vi "Calcualte B Matrix.vi"(6 "Tag ID":i32, 9 "Camera intrinsic matrix (K^-1)":dbl[][](array[numeric]), 10 "Homography H":T1) -> (0 "t Translation Vector":dbl[](array[numeric]), 1 "R Rotation Matrix (final)":T1 format="%#_6f", 2 "B Matrix":dbl[][](array[numeric]))   [LabVIEW 2025]
uses:
  <vilib>/Analysis/Matrix/Datatypes/RealMatrix.ctl
  <vilib>/Analysis/baseanly.llb/Real A x B.vi
  <vilib>/Analysis/baseanly.llb/Real Determinant.vi
  <vilib>/Analysis/7linalg.llb/Real SVD Decomposition.vi
  <vilib>/Analysis/NI_AALPro.lvlib
  <vilib>/Analysis/NI_AALBase.lvlib
  <vilib>/Analysis/Matrix/NI_Matrix.lvlib
panel:
  out "Matrix V":T1
  out "detR":dbl format="%.6f"
  out "detR_temp":dbl format="%.6f"
  out "R^tR":T1 format="%#.3f"
  out "v^t":T1 format="%#_6f"
  out "b1 lambda":dbl
  out "R Matrix":dbl[][](array[numeric])
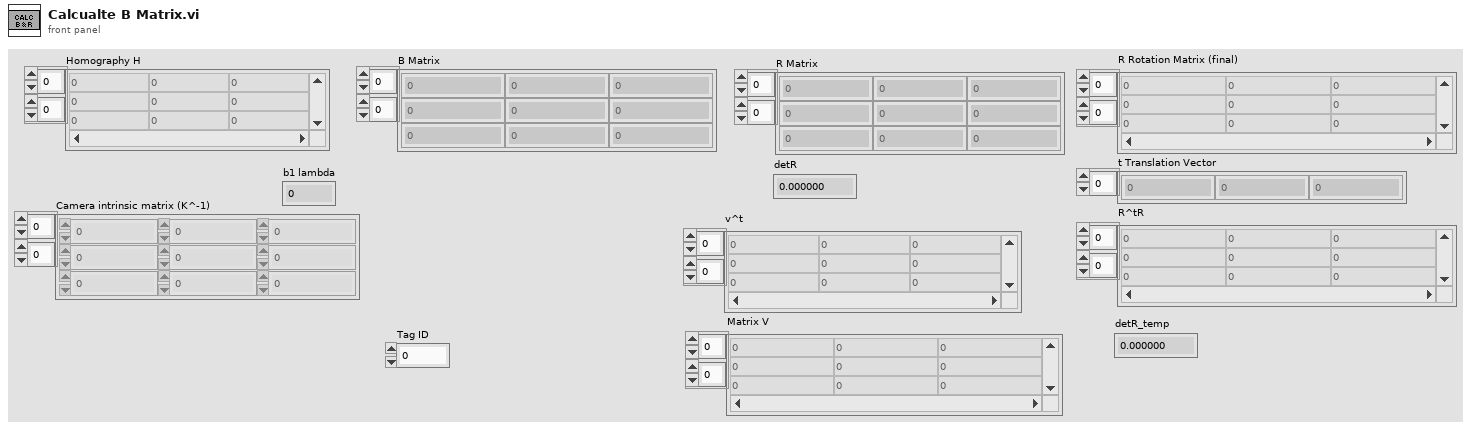
[diagram p1: front panel]
types:
  T1 = typedef "NI_Matrix.lvlib/RealMatrix.ctl" = dbl[][]
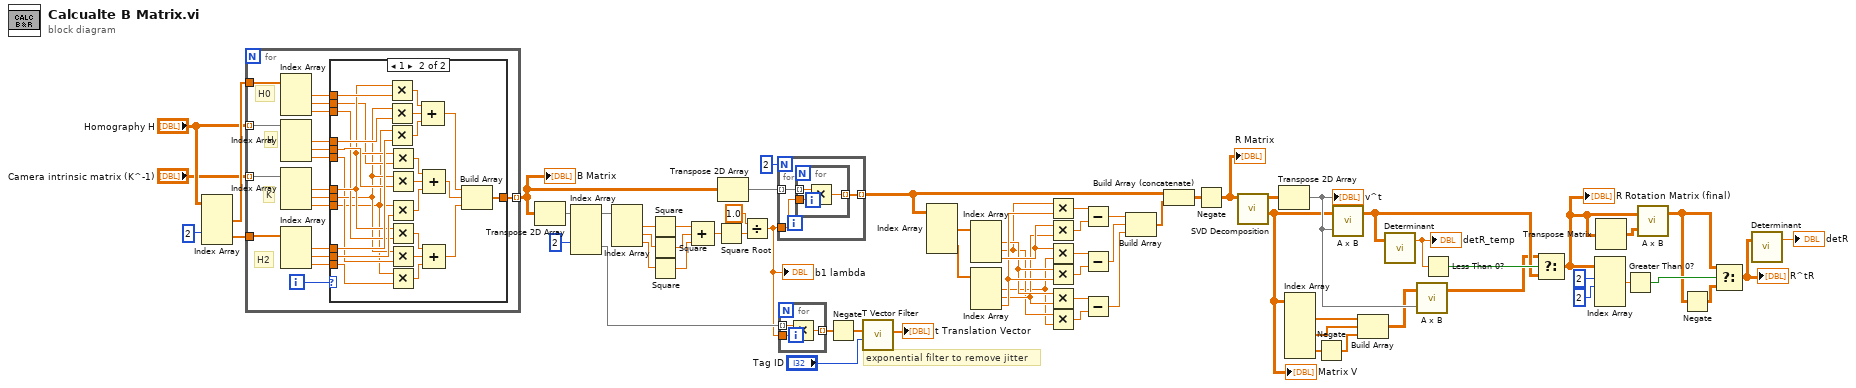
[diagram p0: block diagram]
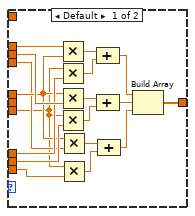
[diagram p2: hidden frame]
diagram:
  # "exponential filter to remove jitter"
  n1 = Index Array(array="Homography H", index (row) #2=2 ("index (row)")) -> (element #1=w69:dbl[], element #2=w68:dbl[])  [unwired: 3 in]
  n2 = for {
    tunnel: "Homography H" -> [w86] mode=indexing
    tunnel: "Camera intrinsic matrix (K^-1)" -> [w87] mode=indexing
    tunnel: w68 -> [w83]
    tunnel: [w76] -> w63 mode=indexing
    tunnel: w69 -> [w73]
    i -> [w75]
    # "H0"
    # "H2"
    # "K"
    # "H"
    n3 = Index Array(array=w73) -> (element #1=w72:dbl, element #2=w71:dbl, element #3=w70:dbl)  [unwired: 3 in]
    n4 = Index Array(array=w86) -> (element #1=w85:dbl, element #2=w84:dbl, element #3=w79:dbl)  [unwired: 3 in]
    n5 = Index Array(array=w87) -> (element #1=w80:dbl, element #2=w74:dbl, element #3=w78:dbl)  [unwired: 3 in]
    n6 = Index Array(array=w83) -> (element #1=w82:dbl, element #2=w81:dbl, element #3=w77:dbl)  [unwired: 3 in]
    n7 = case shown="1" w75 {
      tunnel: w85 -> [w101 w127]
      tunnel: w84 -> [w100 w119]
      tunnel: w82 -> [w99 w125]
      tunnel: w81 -> [w98 w117]
      tunnel: w80 -> [w95 w113]
      tunnel: w79 -> [w94 w108]
      tunnel: w78 -> [w93 w107]
      tunnel: w77 -> [w92 w106]
      tunnel: [w88 w130] -> w76
      tunnel: w74 -> [_ w109]
      tunnel: w72 -> [_ w129]
      tunnel: w71 -> [_ w112]
      tunnel: w70 -> [_ w110]
      frame Default {
        n8 = Multiply(x=w101, y=w95) -> (x*y=w105:dbl)
        n9 = Multiply(x=w93, y=w99) -> (x*y=w104:dbl)
        n10 = Multiply(x=w95, y=w100) -> (x*y=w103:dbl)
        n11 = Multiply(x=w93, y=w98) -> (x*y=w102:dbl)
        n12 = Multiply(x=w95, y=w94) -> (x*y=w96:dbl)
        n13 = Multiply(x=w93, y=w92) -> (x*y=w97:dbl)
        n14 = Compound Arithmetic op=ADD(w105, w104) -> (w91:dbl)
        n15 = Compound Arithmetic op=ADD(w103, w102) -> (w90:dbl)
        n16 = Compound Arithmetic op=ADD(w96, w97) -> (w89:dbl)
        n17 = Build Array(w91, w90, w89) -> (w88:dbl[])
      }
      frame 1 {
        n18 = Multiply(x=w113, y=w129) -> (x*y=w128:dbl)
        n19 = Multiply(x=w109, y=w127) -> (x*y=w126:dbl)
        n20 = Multiply(x=w107, y=w125) -> (x*y=w124:dbl)
        n21 = Multiply(x=w113, y=w112) -> (x*y=w120:dbl)
        n22 = Multiply(x=w109, y=w119) -> (x*y=w121:dbl)
        n23 = Multiply(x=w107, y=w117) -> (x*y=w122:dbl)
        n24 = Multiply(x=w113, y=w110) -> (x*y=w116:dbl)
        n25 = Multiply(x=w109, y=w108) -> (x*y=w115:dbl)
        n26 = Multiply(x=w107, y=w106) -> (x*y=w114:dbl)
        n27 = Compound Arithmetic op=ADD(w128, w126, w124) -> (w123:dbl)
        n28 = Compound Arithmetic op=ADD(w120, w121, w122) -> (w118:dbl)
        n29 = Compound Arithmetic op=ADD(w116, w115, w114) -> (w111:dbl)
        n30 = Build Array(w123, w118, w111) -> (w130:dbl[])
      }
    }
  }
  "B Matrix" <- w63
  n31 = Transpose 2D Array(2D array=w63) -> (transposed array=w64:dbl[][])
  n32 = Index Array(array=w64, index (row) #2=2 ("index (row)")) -> (element #1=w32:dbl[], element #2=w30:dbl[])  [unwired: 3 in]
  n33 = Index Array(array=w32) -> (element #1=w60:dbl, element #2=w59:dbl, element #3=w58:dbl)  [unwired: 3 in]
  n34 = Square(x=w60) -> (x^2=w57:dbl)
  n35 = Square(x=w59) -> (x^2=w56:dbl)
  n36 = Square(x=w58) -> (x^2=w55:dbl)
  n37 = Compound Arithmetic op=ADD(w57, w56, w55) -> (w54:dbl)
  n38 = Square Root(x=w54) -> (sqrt(x)=w52:dbl)
  n39 = Transpose 2D Array(2D array=w63) -> (transposed array=w62:dbl[][])
  n40 = Divide(x=1.0, y=w52) -> (x/y=w29:dbl)
  "b1 lambda" <- w29
  n41 = for {
    N: 2 -> [_]
    tunnel: w62 -> [w133] mode=indexing
    tunnel: w29 -> [w132]
    tunnel: [w131] -> w51 mode=indexing
    n42 = for {
      tunnel: w133 -> [w136] mode=indexing
      tunnel: w132 -> [w135]
      tunnel: [w134] -> w131 mode=indexing
      n43 = Multiply(x=w136, y=w135) -> (x*y=w134:dbl)
    }
  }
  n44 = for {
    tunnel: w30 -> [w138] mode=indexing
    tunnel: w29 -> [w139]
    tunnel: [w137] -> w28 mode=indexing
    n45 = Multiply(x=w138, y=w139) -> (x*y=w137:dbl)
  }
  n46 = Negate(x=w28) -> (-x=w3:dbl[])
  n47 = call "T Vector Filter.vi"("Tag ID"="Tag ID", "t Translation Vector"=w3) -> ("t Translation Vector filtered"=→"t Translation Vector":dbl[])  [unwired: 9 in]
  n48 = Index Array(array=w51) -> (element #1=w50:dbl[], element #2=w49:dbl[])  [unwired: 4 in]
  n49 = Index Array(array=w50) -> (element #1=w40:dbl, element #2=w38:dbl, element #3=w44:dbl)  [unwired: 3 in]
  n50 = Index Array(array=w49) -> (element #1=w37:dbl, element #2=w39:dbl, element #3=w43:dbl)  [unwired: 3 in]
  n51 = Multiply(x=w38, y=w43) -> (x*y=w48:dbl)
  n52 = Multiply(x=w44, y=w39) -> (x*y=w47:dbl)
  n53 = Multiply(x=w44, y=w37) -> (x*y=w45:dbl)
  n54 = Multiply(x=w40, y=w43) -> (x*y=w46:dbl)
  n55 = Multiply(x=w40, y=w39) -> (x*y=w41:dbl)
  n56 = Multiply(x=w38, y=w37) -> (x*y=w42:dbl)
  n57 = Subtract(x=w48, y=w47) -> (x-y=w36:dbl)
  n58 = Subtract(x=w45, y=w46) -> (x-y=w35:dbl)
  n59 = Subtract(x=w41, y=w42) -> (x-y=w34:dbl)
  n60 = Build Array(w36, w35, w34) -> (w33:dbl[])
  n61 = Build Array (concatenate)(w51, w33) -> (w26:dbl[][])
  n62 = Negate(x=w26) -> (-x=w24:dbl[][])
  "R Matrix" <- w24
  n63 = call-poly <vilib>:"SVD Decomposition.vi"("A"=w24) -> ("Matrix V"=w6:T1, "Matrix U"=w27:T1)  [unwired: 6 in, 3 out]
  "Matrix V" <- w6
  n64 = Transpose 2D Array(2D array=w27) -> (transposed array=w16:T1)
  "v^t" <- w16
  n65 = Index Array(array=w6) -> (element #1=w10:dbl[], element #2=w9:dbl[], element #3=w8:dbl[])  [unwired: 6 in]
  n66 = Negate(x=w8) -> (-x=w7:dbl[])
  n67 = call-poly <vilib>:"A x B.vi"("B"=w16, "A"=w6) -> ("A x B"=w14:T1)  [unwired: 1 out]
  n68 = Build Array(w10, w9, w7) -> (w5:dbl[][])
  n69 = call-poly <vilib>:"Determinant.vi"("Input Matrix"=w14) -> ("determinant"=w17:dbl)  [unwired: 1 in, 1 out]
  "detR_temp" <- w17
  n70 = call-poly <vilib>:"A x B.vi"("B"=w16, "A"=w5) -> ("A x B"=w4:T1)  [unwired: 1 out]
  n71 = Less Than 0?(x=w17) -> (x < 0?=w15:bool)
  n72 = Select(t=w4, s=w15, f=w14) -> (s? t:f=w13:T1)
  "R Rotation Matrix (final)" <- w13
  n73 = Index Array(array=w13, index (row) #1=2 ("index (row)"), index (col) #1=2 ("disabled index (col)")) -> (element #1=w21:dbl)  [unwired: 2 in, 1 out]
  n74 = Transpose Matrix(1:w13) -> (0:w25:T1)
  n75 = Greater Than 0?(x=w21) -> (x > 0?=w20:bool)
  n76 = call-poly <vilib>:"A x B.vi"("B"=w25, "A"=w13) -> ("A x B"=w19:T1)  [unwired: 1 out]
  n77 = Negate(x=w19) -> (-x=w18:T1)
  n78 = Select(t=w19, s=w20, f=w18) -> (s? t:f=w11:T1)
  "R^tR" <- w11
  n79 = call-poly <vilib>:"Determinant.vi"("Input Matrix"=w11) -> ("determinant"=→"detR":dbl)  [unwired: 1 in, 1 out]
